vi "ge_EditString.vi"(4 "CellSize":T2, 6 "ActiveCellPos":T1, 7 "String":string, 8 "error in":errorcluster, 11 "FP Ctrl":T3) -> (0 "error out":errorcluster, 1 "Discard?":bool)   [LabVIEW 2012]
uses:
  Custom Ctrls/ge_FPCtrlRefLabel.ctl
  <vilib>/Utility/miscctls.llb/LVBoundsTypeDef.ctl
  <vilib>/Utility/miscctls.llb/LVPositionTypeDef.ctl
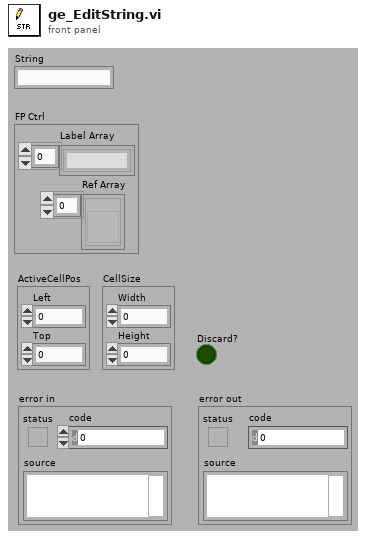
[diagram p1: front panel]
types:
  T1 = typedef "LVPositionTypeDef.ctl" = cluster{"Left":i32, "Top":i32}
  T2 = typedef "LVBoundsTypeDef.ctl" = cluster{"Width":u32, "Height":u32}
  T3 = typedef "ge_FPCtrlRefLabel.ctl" = cluster{"Label Array":string[], "Ref Array":refnum<vi>[]}
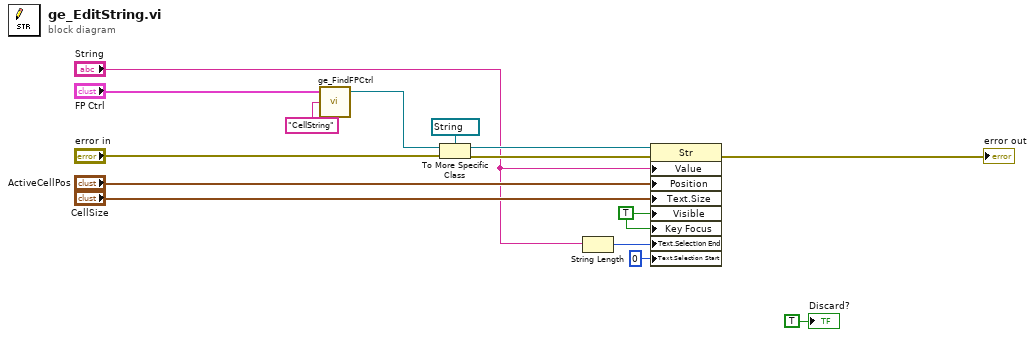
[diagram p0: block diagram]
diagram:
  w2 = TRUE ("Visible")
  n1 = call "ge_FindFPCtrl.vi"("Ctrl Name"="CellString" ("Name"), "FP Ctrl"="FP Ctrl") -> ("Ctrl Ref"=w15:refnum<vi>)  [unwired: 3 in]
  n2 = To More Specific Class(target class=refnum<vi> refnum ("reference"), reference=w15, error in="error in") -> (specific class reference=w12:refnum<vi>, error out=w13:errorcluster)
  n3 = String Length(string="String") -> (length=w3:i32)
  n4 = property on="Property Node" class="Str"(reference=w12, error in=w13, "Value"="String", "Position"="ActiveCellPos", "Text.Size"="CellSize", "Visible"=w2, "Key Focus"=w2, "Text.Selection End"=w3, "Text.Selection Start"=u32 0 ("Text.Selection:Start")) -> (error out=→"error out":errorcluster)  [unwired: 1 out]
  "Discard?" <- TRUE ("Discard?")
